vi "sv_Check for df Change.vi"(8 "error in (no error)":errorcluster, 11 "power spectrum":cluster{"f0":dbl, "df":dbl, "Spectrum":dbl[]} {"Spectrum" format="%.2f"; "df" format="%.2f"; "f0" format="%.2f"}) -> (0 "error out":errorcluster, 1 "param has changed":bool, 3 "dup power spectrum":cluster{"f0":dbl, "df":dbl, "Spectrum":dbl[]} {"Spectrum" format="%.2f"; "df" format="%.2f"; "f0" format="%.2f"})   [LabVIEW 2017]
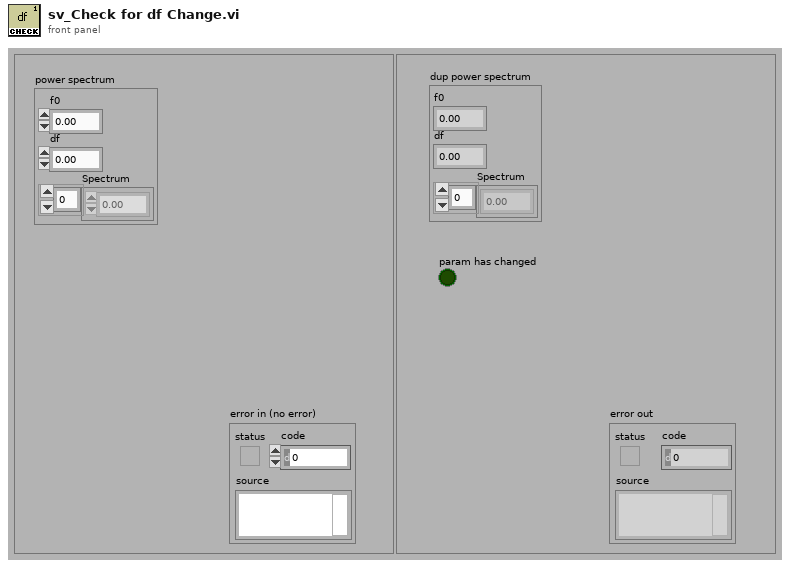
[diagram p1: front panel]
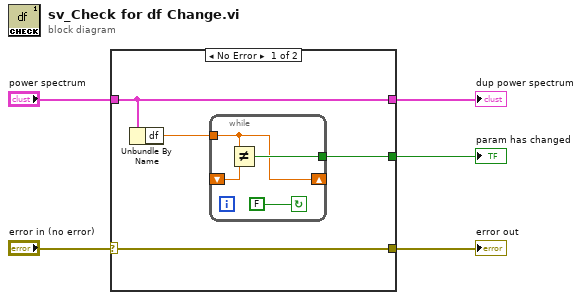
[diagram p0: block diagram]
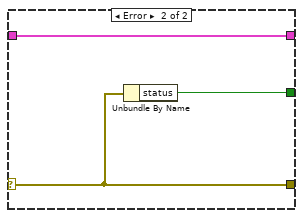
[diagram p2: hidden frame]
diagram:
  n1 = case shown="No Error" "error in (no error)" {
    selector: "error in (no error)" -> [w6 w15]
    tunnel: "power spectrum" -> [w8 w16]
    tunnel: [w6 w15] -> w4
    tunnel: [w8 w16] -> w2
    tunnel: [w7 w14] -> w1
    frame No Error {
      n2 = Unbundle By Name(w8) -> ("df"=w9:dbl)
      n3 = while {
        tunnel: [w12] -> w7
        tunnel: w9 -> [w10]
        shift-left: _ -> [w11]
        shift-right: [w10] -> _
        stop <- FALSE continue-if-true
        n4 = Not Equal?(x=w10, y=w11) -> (x != y?=w12:bool)
      }
    }
    frame Error {
      n5 = Unbundle By Name(w15) -> ("status"=w14:bool)
    }
  }
  "error out" <- w4
  "dup power spectrum" <- w2
  "param has changed" <- w1
